vi "ServerRefnum.vi"(3 "error in (no error)":errorcluster) -> (16 "OPC UA server refnum":refnum<k21>, 17 "error out":errorcluster)   [LabVIEW 2014, in "OPCUA Server(UtilityMode)(dev).lvlib"]
uses:
  OPCUA Server(UtilityMode)(dev).lvlib
  _op(server).ctl
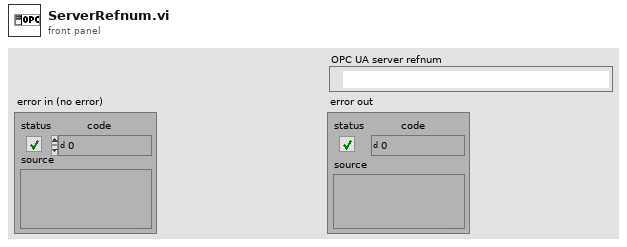
[diagram p1: front panel]
types:
  T1 = typedef "OPCUA Server(UtilityMode)(dev).lvlib/_op(server).ctl" = enum16{"Create Server", "Start Server", "Get Server Refnum", "Stop Server", "Close Server"}
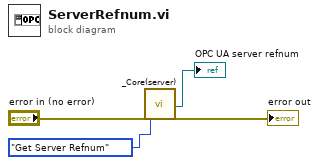
[diagram p0: block diagram]
diagram:
  n1 = call "_Core(server).vi"("error in (no error)"="error in (no error)", "Op"=_op(server)."Get Server Refnum") -> ("OPC UA server refnum"=→"OPC UA server refnum":refnum<k21>, "error out"=→"error out":errorcluster)  [unwired: 21 in, 3 out]
